vi "Set Error Reporting.vi"(8 "error in (no error)":errorcluster, 10 "Error Reporting":T1, 11 "Session in":refnum<class "Session.lvclass">) -> (0 "error out":errorcluster, 3 "Session out":refnum<class "Session.lvclass">)   [LabVIEW 2020, in "CTI.lvlib" / "Session.lvclass"]
uses:
  Session.lvclass
  Session.lvclass/Session.ctl
  Error Reporting.ctl
  CTI.lvlib
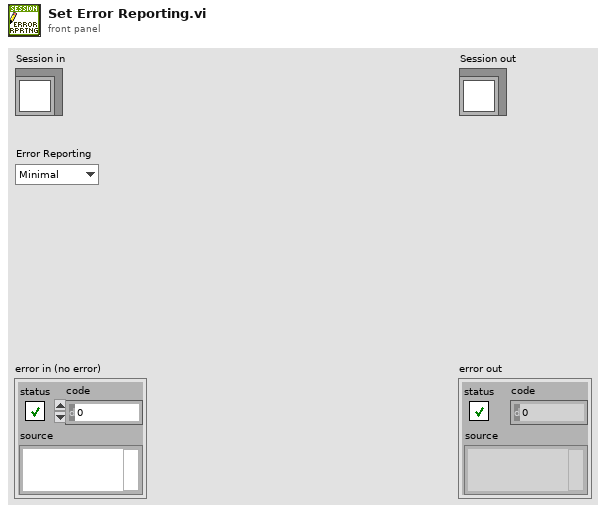
[diagram p1: front panel]
types:
  T1 = typedef "CTI.lvlib/Error Reporting.ctl" = enum16{"Minimal", "Moderate", "Full"}
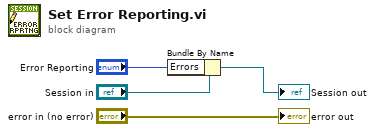
[diagram p0: block diagram]
diagram:
  n1 = Bundle By Name(cluster="Session in", "Errors"="Error Reporting") -> (→"Session out":refnum<class "Session.lvclass">)
  "error out" <- "error in (no error)"
